vi "Drive Controller.vi"(8 "error in":errorcluster) -> ()   [LabVIEW 2015]
doc: "This VI executes continuously carrying out the current operation and responding to updates or new operation requests. It will often contain the timing or control code that is difficult to place directly in TeleOp. This VI generally opens all sensors and motors and isolates the rest of the robot code from knowing implementation details of how the operations are carried out."
uses:
  Drive Setpoints.ctl
  Drive Operations.ctl
  <vilib>/Rock Robotics/WPI/SafetyOutput/WPI_SafetyOutputConfigMenu.ctl
  <vilib>/Rock Robotics/SystemInterfaces/DIO/FPGA_DIOChannel.ctl
  <vilib>/Rock Robotics/SystemInterfaces/AI/FPGA_AIGyroChannel.ctl
  <vilib>/Rock Robotics/WPI/Counter/WPI_CounterDigitalInputToDigitalSource.vi
  <vilib>/Rock Robotics/WPI/Gyro/WPI_GyroAnalogOpen.vi
  <vilib>/Rock Robotics/WPI/RobotDrive/WPI_RobotDriveOpen4MotorWithCANTalonSRX.vi
panel:
  out "Numeric":i64
  out "Setpoints":T1(graph)
  out "Current\nCmd":string
  # "Tip: It may be helpful to observe inputs and sensor values.\nYou may also want to display tuning or debugging controls."
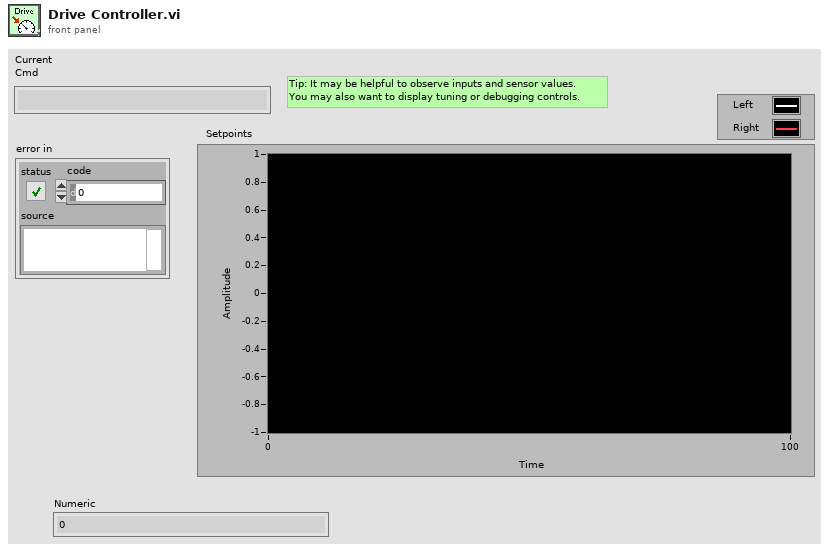
[diagram p1: front panel]
types:
  T1 = cluster{"Left Setpoint":dbl, "Right Setpoint":dbl}
  T2 = typedef "FPGA_AIGyroChannel.ctl" = enum8{"AI 0", "AI 1", "Invalid"}
  T3 = typedef "FPGA_DIOChannel.ctl" = enum8{"DIO 0", "DIO 1", "DIO 2", "DIO 3", "DIO 4", "DIO 5", "DIO 6", "DIO 7", "DIO 8", "DIO 9", "DIO MXP 0", "DIO MXP 1", "DIO MXP 2", "DIO MXP 3", "DIO MXP 4", "DIO MXP 5", "DIO MXP 6", "DIO MXP 7", "DIO MXP 8", "DIO MXP 9", "DIO MXP 10", "DIO MXP 11", "DIO MXP 12", "DIO MXP 13", "DIO MXP 14", "DIO MXP 15", "Invalid"}
  T4 = typedef "WPI_SafetyOutputConfigMenu.ctl" = enum16{"Enable", "Disable"}
  T5 = typedef "Drive Setpoints.ctl" = cluster{"Operation":T6, "Left Setpoint":dbl, "Right Setpoint":dbl, "Duration":dbl, "Distance":dbl}
  T6 = typedef "Drive Operations.ctl" = enum16{"Reserve", "Read Current", "Immediate", "Drive for Time", "Drive for Distance", "Drive With Gyro", "visiontrack"}
  T7 = typedef "WPI_DigitalInputDevRef.ctl" = cluster{"DevStatus":errorcluster, "DIO Channel":T3}
  T8 = typedef "WPI_RobotDriveDevRef.ctl" = cluster{"DevStatus":errorcluster, "Motors[]":T9[], "Square Inputs":bool, "Max Output":dbl}
  T9 = typedef "WPI_MotorControlDeviceRef.ctl" = cluster{"DeviceStatus":errorcluster, "Type":T10, "PWM":cluster{"PWM Channel":T11, "DeadBand":T12}, "CAN":cluster{"Device Number":u8, "Control Mode":T13, "Semaphore":T14, "Max Vout":dbl, "TalonSRX Control Mode":T15}, "Invert":bool}
  T10 = typedef "WPI_MotorControlType.ctl" = enum16{"PWM", "CAN", "CANTalonSRX"}
  T11 = typedef "FPGA_DIOPWMChannel.ctl" = enum8{"PWM 0", "PWM 1", "PWM 2", "PWM 3", "PWM 4", "PWM 5", "PWM 6", "PWM 7", "PWM 8", "PWM 9", "PWM MXP 0", "PWM MXP 1", "PWM MXP 2", "PWM MXP 3", "PWM MXP 4", "PWM MXP 5", "PWM MXP 6", "PWM MXP 7", "PWM MXP 8", "PWM MXP 9", "Invalid"}
  T12 = typedef "WPI_PWMDeadband.ctl" = cluster{"Name":string, "maxPositivePwm":i32, "minPositivePwm":i32, "centerPwm":i32, "maxNegativePwm":i32, "minNegativePwm":i32, "angularRange":u16}
  T13 = typedef "WPI_CANJaguar_ControlMode.ctl" = enum8{"Percent VBus", "Current", "Speed", "Position", "Voltage"}
  T14 = typedef "Semaphore RefNum" = refnum<k1>
  T15 = typedef "WPI_CANTalonSRX_APIControlMode.ctl" = enum8{"Percent VBus", "Speed", "Position", "Slave", "Unchanged / Invalid", "Voltage Compensation", "Current", "Motion Profile"}
  T16 = typedef "FPGA_CounterEncoderSourceConvertionLVSourceType.ctl" = cluster{"DevStatus":errorcluster, "AnalogTriggerMode?":bool, "DigitalMode":cluster{"DIO Channel":T17}, "AnalogTriggerMode":cluster{"AnalogTriggerIndex":T18, "OutputType":T19}}
  T17 = typedef "FPGA_DIODigitalSourceChannel.ctl" = enum8{"DIO 0", "DIO 1", "DIO 2", "DIO 3", "DIO 4", "DIO 5", "DIO 6", "DIO 7", "DIO 8", "DIO 9", "DIO MXP 0", "DIO MXP 1", "DIO MXP 2", "DIO MXP 3", "DIO MXP 4", "DIO MXP 5", "DIO MXP 6", "DIO MXP 7", "DIO MXP 8", "DIO MXP 9", "DIO MXP 10", "DIO MXP 11", "DIO MXP 12", "DIO MXP 13", "DIO MXP 14", "DIO MXP 15", "Disabled"}
  T18 = typedef "FPGA_AnalogTriggerIndex.ctl" = enum8{"Trig 0", "Trig 1", "Trig 2", "Trig 3", "Trig 4", "Trig 5", "Trig 6", "Trig 7", "Invalid"}
  T19 = typedef "FPGA_AnalogTriggerOutType.ctl" = enum16{"InWindow", "TriggerState", "Rising", "Falling"}
  T20 = typedef "WPI_EncoderDevRef.ctl" = cluster{"DevStatus":errorcluster, "EncoderIndex":T21, "CounterIndex":T22, "DistancePerCount":dbl, "Decoding Type":T23}
  T21 = typedef "FPGA_EncoderIdx.ctl" = enum8{"Enc 0", "Enc 1", "Enc 2", "Enc 3", "Enc 4", "Enc 5", "Enc 6", "Enc 7", "Invalid"}
  T22 = typedef "FPGA_CounterCtrSystemIndex.ctl" = enum8{"Ctr 0", "Ctr 1", "Ctr 2", "Ctr 3", "Ctr 4", "Ctr 5", "Ctr 6", "Ctr 7", "Invalid"}
  T23 = typedef "WPI_EncoderType.ctl" = enum16{"1x", "2x", "4x"}
  T24 = typedef "WPI_GyroDevRef.ctl" = cluster{"DevStatus":errorcluster, "Analog Channel":T25, "Offset":dbl, "Gain (VoltsPerDegree/Second)":dbl, "Gyro Type":enum16{"Analog", "XRS450"}, "Handle":i32, "SPI Bus":T26, "Device Found":bool, "Sample Rate":dbl, "Calibrate On Open":bool}
  T25 = typedef "FPGA_AIChannel.ctl" = enum8{"AI 0", "AI 1", "AI 2", "AI 3", "AI MXP 0", "AI MXP 1", "AI MXP 2", "AI MXP 3", "Invalid"}
  T26 = typedef "spi_bus.ctl" = enum16{"SPI On-Board, CS0", "SPI On-Board, CS1", "SPI On-Board, CS2", "SPI On-Board, CS3", "SPI MXP", "Invalid"}
  T27 = typedef "Command Status Info.ctl" = cluster{"Name":string, "Status":T28, "notifier out":T29}
  T28 = typedef "Completion Status.ctl" = enum16{"Successful", "Aborted", "Incomplete"}
  T29 = typedef "Completion Notifier.ctl" = refnum<notifier>
  T30 = cluster{"SubSystem Data":T5, cluster{"Start Time (ms)":u32, "Iterations":i32}, cluster{"Command Info":T27, "Description":string, "SubSystem Data":T5, "notifier out":refnum<notifier>, "Subsystem Name":string}}
  T31 = cluster{"SubSystem Data":T5, cluster{"Start Time (ms)":u32, "Iterations":i32}, "Default Command Arguments":cluster{"Command Info":T27, "Description":string, "SubSystem Data":T5, "notifier out":refnum<notifier>, "Subsystem Name":string}}
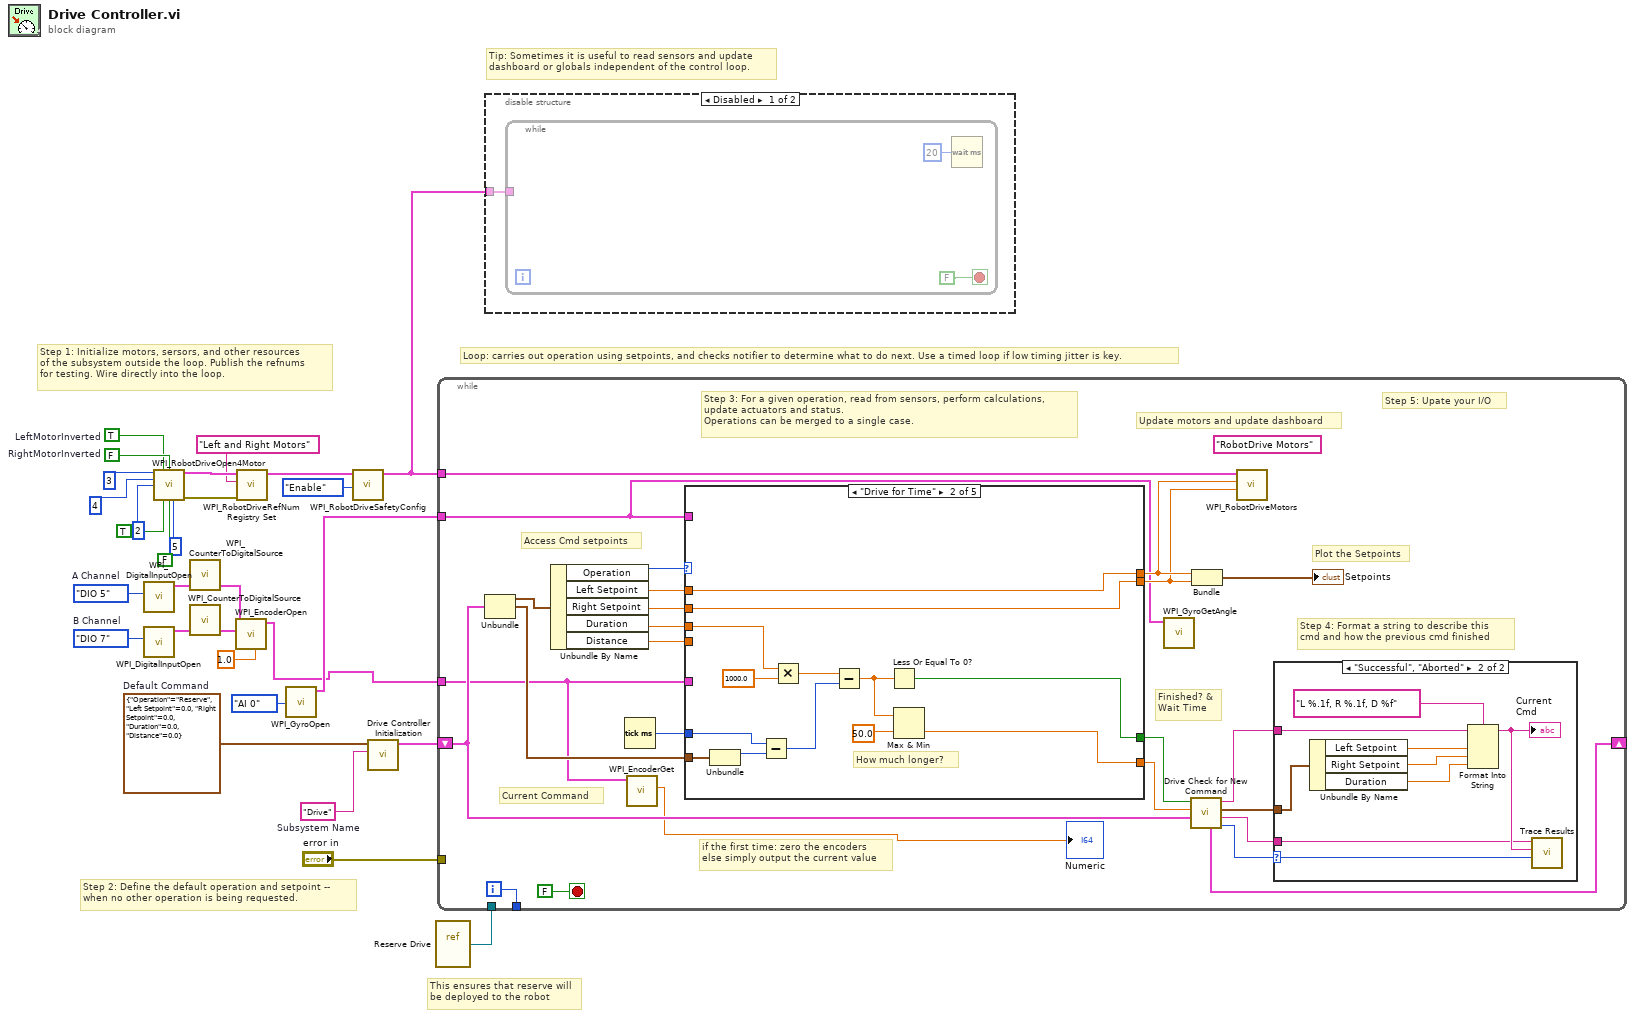
[diagram p0: block diagram]
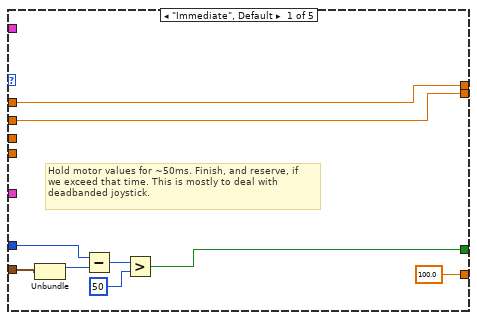
[diagram p4: hidden frame]
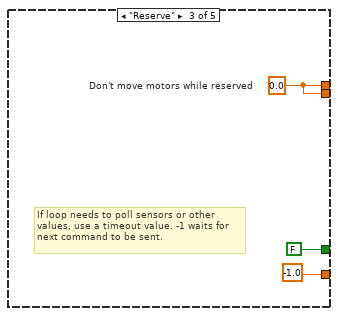
[diagram p5: hidden frame]
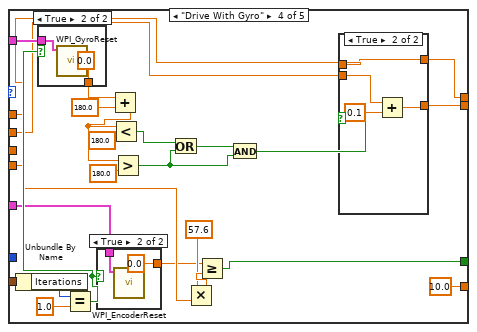
[diagram p6: hidden frame]
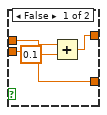
[diagram p7: hidden frame]
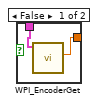
[diagram p8: hidden frame]
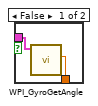
[diagram p9: hidden frame]
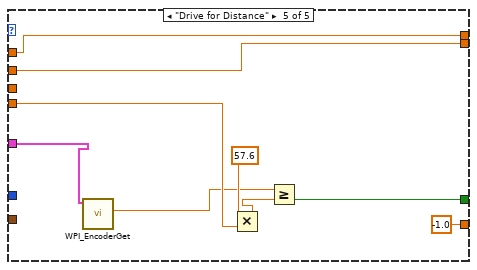
[diagram p10: hidden frame]
diagram:
  w14 = FPGA_DIOChannel."DIO 7"  # B Channel
  w13 = FPGA_DIOChannel."DIO 5"  # A Channel
  w24 = TRUE  # LeftMotorInverted
  w25 = FALSE  # RightMotorInverted
  w28 = T5 {"Operation"=enum."Reserve", "Left Setpoint"=0.0, "Right Setpoint"=0.0, "Duration"=0.0, "Distance"=0.0}  # Default Command
  w29 = "Drive"  # Subsystem Name
  # "This ensures that reserve will\nbe deployed to the robot"
  # "Tip: Sometimes it is useful to read sensors and update\ndashboard or globals independent of the control loop."
  # "Step 2: Define the default operation and setpoint --\nwhen no other operation is being requested."
  # "Step 1: Initialize motors, sersors, and other resources\nof the subsystem outside the loop. Publish the refnums\nfor testing. Wire directly into the loop."
  # "Loop: carries out operation using setpoints, and checks notifier to determine what to do next. Use a timed loop if low timing jitter is key."
  n1 = call <vilib>:"WPI_DigitalInputOpen.vi"("DIO Channel"=w13) -> ("DigitalInputDevRef"=w10:T7)  [unwired: 1 in, 9 out]
  n2 = call <vilib>:"WPI_DigitalInputOpen.vi"("DIO Channel"=w14) -> ("DigitalInputDevRef"=w11:T7)  [unwired: 1 in, 9 out]
  n3 = call-poly <vilib>:"WPI_RobotDriveOpen4Motor.vi"("Rear Left Motor"=u8 3 ("Left Motor"), "Rear Left Motor Inverted"=w24, "Rear Right Motor Inverted"=w25, "Rear Right Motor"=u8 4 ("Left Motor"), "Front Left Motor"=u8 2, "Front Right Motor"=u8 5, "Front Left Motor Inverted"=TRUE, "Front Right Motor Inverted"=FALSE) -> ("RobotDriveDevRef"=w23:T8, "error out"=w21:errorcluster)  [unwired: 6 in]
  n4 = call-poly <vilib>:"WPI_CounterToDigitalSource.vi"("DigitalInputDevRef"=w10) -> ("Digital Source"=w9:T16)  [unwired: 6 out]
  n5 = call-poly <vilib>:"WPI_CounterToDigitalSource.vi"("DigitalInputDevRef"=w11) -> ("Digital Source"=w12:T16)  [unwired: 6 out]
  n6 = call <vilib>:"WPI_EncoderOpen.vi"("DistancePerCount"=1.0, "BSource"=w12, "ASource"=w9) -> ("EncoderDevRef"=w1:T20)  [unwired: 5 in, 3 out]
  n7 = call <vilib>:"WPI_RobotDriveRefNum Registry Set.vi"("error in (no error)"=w21, "refnum name"="Left and Right Motors", "RobotDriveDevRef"=w23) -> ("RobotDriveDevRef"=w20:T8)  [unwired: 1 in, 7 out]
  n8 = call-poly <vilib>:"WPI_GyroOpen.vi"("Analog Channel"=FPGA_AIGyroChannel."AI 0") -> ("GyroDevRef"=w7:T24)  [unwired: 8 in, 2 out]
  n9 = call <vilib>:"WPI_RobotDriveSafetyConfig.vi"("mode"=WPI_SafetyOutputConfigMenu."Enable", "RobotDriveDevRef"=w20) -> ("RobotDriveDevRef"=w18:T8)  [unwired: 8 in, 1 out]
  n10 = call "Drive Controller Initialization.vi"("Subsystem Name"=w29, "Default Command"=w28) -> ("output cluster"=w16:T30)  [unwired: 9 in]
  n11 = vi-ref "Reserve Drive.vi"() -> (w15:refnum<vi>)
  n12 = while {
    shift-right: [w41] -> _
    shift-left: w16 -> [w34]
    tunnel: [w53] -> _
    tunnel: w18 -> [w49]
    tunnel: "error in" -> [_]
    tunnel: w15 -> [_]
    tunnel: w7 -> [w32]
    tunnel: w1 -> [w31]
    i -> [w53]
    stop <- FALSE stop-if-true
    (unwired) "RobotDrive Motors" ("Name")
    # "if the first time: zero the encoders\nelse simply output the current value"
    # "Step 5: Upate your I/O"
    # "Step 4: Format a string to describe this\ncmd and how the previous cmd finished"
    # "Current Command"
    # "Update motors and update dashboard"
    # "Plot the Setpoints"
    # "Access Cmd setpoints"
    # "Finished? &\nWait Time"
    # "Step 3: For a given operation, read from sensors, perform calculations,\nupdate actuators and status.\nOperations can be merged to a single case."
    n13 = Unbundle(w34) -> ("SubSystem Data"=w48:T5, w35:cluster{"Start Time (ms)":u32, "Iterations":i32})  [unwired: 1 out]
    n14 = Unbundle By Name(w48) -> ("Operation"=w47:T6, "Left Setpoint"=w46:dbl, "Right Setpoint"=w45:dbl, "Duration"=w44:dbl, "Distance"=w33:dbl)
    n15 = Tick Count (ms)() -> (millisecond timer value=w43:u32)
    n16 = call <vilib>:"WPI_EncoderGet.vi"("EncoderDevRef"=w31) -> ("Distance"=→"Numeric":dbl)  [unwired: 5 in, 5 out]
    n17 = case shown="\"Drive for Time\"" w47 {
      tunnel: [100.0 w73 -1.0 10.0 -1.0] -> w40
      tunnel: [w65 w80 FALSE ("ignore previous (F)") w94 w135] -> w39
      tunnel: w35 -> [w64 w82 _ w113 _]
      tunnel: [w71 w79 w86 w103 w133] -> w51
      tunnel: [w70 w78 w86 w102 w132] -> w50
      tunnel: w46 -> [w71 w79 _ w110 w133]
      tunnel: w45 -> [w70 w78 _ w89 w132]
      tunnel: w44 -> [_ w77 _ _ _]
      tunnel: w43 -> [w66 w76 _ _ _]
      tunnel: w33 -> [_ _ _ w97 w136]
      tunnel: w32 -> [_ _ _ w91 _]
      tunnel: w31 -> [_ _ _ w90 w131]
      frame "Immediate", Default {
        # "Hold motor values for ~50ms. Finish, and reserve, if\nwe exceed that time. This is mostly to deal with\ndeadbanded joystick."
        n18 = Unbundle(w64) -> ("Start Time (ms)"=w67:u32)  [unwired: 1 out]
        n19 = Subtract(x=w66, y=w67) -> (x-y=w68:u32)
        n20 = Greater?(x=w68, y=u8 50 ("Left Motor")) -> (0:w65:bool)
      }
      frame "Drive for Time" {
        # "How much longer?"
        n21 = Unbundle(w82) -> ("Start Time (ms)"=w81:u32)  [unwired: 1 out]
        n22 = Subtract(x=w76, y=w81) -> (x-y=w85:u32)
        n23 = Multiply(x=w77, y=1000.0) -> (x*y=w84:dbl)
        n24 = Subtract(x=w84, y=w85) -> (x-y=w75:dbl)
        n25 = Less Or Equal To 0?(x=w75) -> (x <= 0?=w80:bool)
        n26 = Max & Min(x=w75, y=50.0) -> (min(x,y)=w73:dbl)  [unwired: 1 out]
      }
      frame "Reserve" {
        w86 = 0.0  # Don't move motors while reserved
        # "If loop needs to poll sensors or other\nvalues, use a timeout value. -1 waits for\nnext command to be sent."
      }
      frame "Drive With Gyro" {
        n27 = Unbundle By Name(w113) -> ("Iterations"=w92:i32)
        n28 = Equal?(x=w92, y=1.0) -> (x = y?=w111:bool)
        n29 = case shown="True" w111 {
          tunnel: [w127 0.0 ("Angle")] -> w101
          tunnel: w91 -> [w126 w128]
          frame False {
            n30 = call <vilib>:"WPI_GyroGetAngle.vi"("GyroDevRef"=w126) -> ("Angle"=w127:dbl)  [unwired: 6 in, 4 out]
          }
          frame True {
            n31 = call <vilib>:"WPI_GyroReset.vi"("GyroDevRef"=w128) -> ()  [unwired: 9 in, 2 out]
          }
        }
        n32 = case shown="True" w111 {
          tunnel: [w123 0.0 ("Distance")] -> w95
          tunnel: w90 -> [w122 w124]
          frame False {
            n33 = call <vilib>:"WPI_EncoderGet.vi"("EncoderDevRef"=w122) -> ("Distance"=w123:dbl)  [unwired: 5 in, 5 out]
          }
          frame True {
            n34 = call <vilib>:"WPI_EncoderReset.vi"("EncoderDevRef"=w124) -> ()  [unwired: 9 in, 2 out]
          }
        }
        n35 = Add(x=w101, y=180.0) -> (x+y=w99:dbl)
        n36 = Less?(x=w99, y=180.0) -> (x < y?=w107:bool)
        n37 = Greater?(x=w99, y=180.0) -> (0:w105:bool)
        n38 = Or(x=w107, y=w105) -> (x .or. y?=w106:bool)
        n39 = Multiply(x=57.6, y=w97) -> (x*y=w98:dbl)
        n40 = Greater Or Equal?(x=w95, y=w98) -> (x >= y?=w94:bool)
        n41 = And(x=w106, y=w105) -> (x .and. y?=w104:bool)
        n42 = case shown="True" w104 {
          tunnel: w110 -> [w116 w121]
          tunnel: w89 -> [w117 w119]
          tunnel: [w114 w121] -> w103
          tunnel: [w117 w118] -> w102
          frame False {
            n43 = Add(x=w116, y=0.1) -> (x+y=w114:dbl)
          }
          frame True {
            n44 = Add(x=w119, y=0.1) -> (x+y=w118:dbl)
          }
        }
      }
      frame "Drive for Distance" {
        n45 = call <vilib>:"WPI_EncoderGet.vi"("EncoderDevRef"=w131) -> ("Distance"=w130:dbl)  [unwired: 5 in, 5 out]
        n46 = Multiply(x=57.6, y=w136) -> (x*y=w138:dbl)
        n47 = Greater Or Equal?(x=w130, y=w138) -> (x >= y?=w135:bool)
      }
    }
    n48 = call <vilib>:"WPI_GyroGetAngle.vi"("GyroDevRef"=w32) -> ()  [unwired: 6 in, 5 out]
    n49 = call "Drive Check for New Command.vi"("input cluster"=w34, "Wait time (ms)"=w40, "Finished?"=w39) -> ("Completion"=w42:T28, "Subsystem Name"=w36:string, "SetPoint"=w37:T5, "Initial Trace String"=w38:string, "output cluster"=w41:T31)  [unwired: 4 in]
    n50 = Bundle("Left Setpoint"=w51, "Right Setpoint"=w50) -> (→"Setpoints":T1)  [unwired: 1 in]
    n51 = call <vilib>:"WPI_RobotDriveMotors.vi"("RightSpeed"=w50, "LeftSpeed"=w51, "RobotDriveDevRef"=w49) -> ()  [unwired: 1 in, 8 out]
    n52 = case shown="\"Successful\", \"Aborted\"" w42 {
      selector: w42 -> [_ w63]
      tunnel: w38 -> [_ w58]
      tunnel: w37 -> [_ w59]
      tunnel: w36 -> [_ w55]
      frame "Incomplete", Default {
        # "Continuing current command"
      }
      frame "Successful", "Aborted" {
        # "Report and setup for next command"
        n53 = Unbundle By Name(w59) -> ("Left Setpoint"=w61:dbl, "Right Setpoint"=w62:dbl, "Duration"=w56:dbl)
        n54 = Format Into String(format string="L %.1f, R %.1f, D %f", initial string=w58, w61, w62, w56) -> (resulting string=w57:string)  [unwired: 1 in, 1 out]
        "Current\nCmd" <- w57
        n55 = call <vilib>:"Trace Results.vi"("Status of previous command"=w63, "Description"=w57, "Subsystem"=w55) -> ()  [unwired: 9 in]
      }
    }
  }
  n56 = disable-structure shown="Disabled" {
    disable-tunnel: w18 -> [w139 _]
    frame Disabled {
      n57 = while {
        tunnel: w139 -> [_]
        stop <- FALSE stop-if-true
        n58 = Wait (ms)(milliseconds to wait=u32 20) -> ()  [unwired: 1 out]
      }
    }
    frame Enabled {
    }
  }
